vi "DifficultyValueChange.vi"(8 "error in (no error)":errorcluster, 11 "View in":refnum<class "View.lvclass">) -> (0 "error out":errorcluster, 3 "View out":refnum<class "View.lvclass">)   [LabVIEW 2024, in "GUI.lvlib" / "View.lvclass"]
uses:
  View.lvclass
  TypeDefs/Settings.ctl
  View.lvclass/View.ctl
  Controller/Controller.lvclass
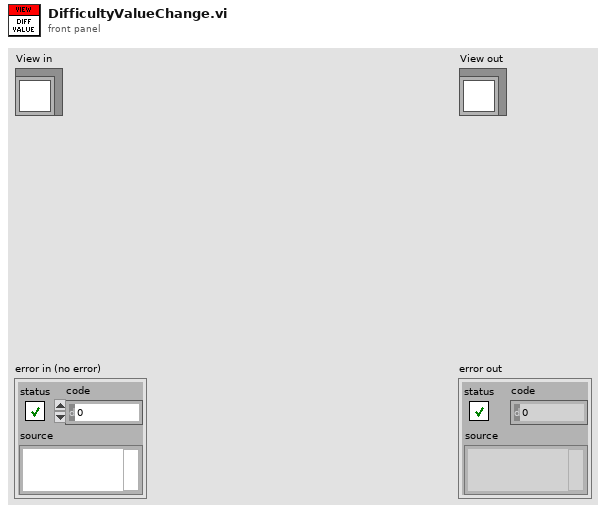
[diagram p1: front panel]
types:
  T1 = typedef "Settings.ctl" = cluster{"Difficulty":i32}
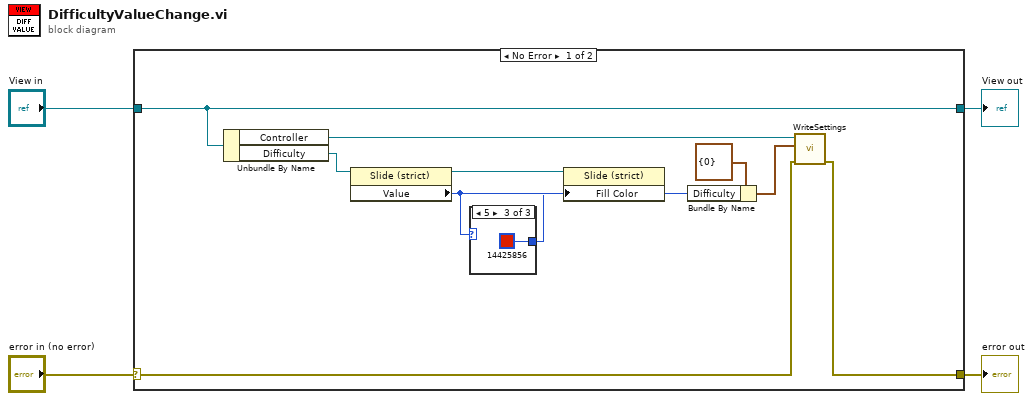
[diagram p0: block diagram]
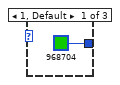
[diagram p2: hidden frame]
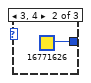
[diagram p3: hidden frame]
diagram:
  n1 = case shown="No Error" "error in (no error)" {
    selector: "error in (no error)" -> [w10 w19]
    tunnel: [w9 w19] -> w3
    tunnel: [w8 w18] -> w1
    tunnel: "View in" -> [w8 w18]
    frame No Error {
      n2 = Unbundle By Name(w8) -> ("Controller"=w14:refnum<class "Controller.lvclass">, "Difficulty"=w13:refnum<vi>)
      n3 = property class="Slide (strict)"(reference=w13) -> (reference out=w7:refnum<vi>, "Value"=w6:i32)  [unwired: 1 in, 1 out]
      n4 = case shown="5" w6 {
        tunnel: [u32 968704 u32 16771626 u32 14425856] -> w5
        frame 1, Default {
        }
        frame 3, 4 {
        }
        frame 5 {
        }
      }
      n5 = property class="Slide (strict)"(reference=w7, "Fill Color"=w5) -> ()  [unwired: 1 in, 2 out]
      n6 = Bundle By Name(cluster=T1 {"Difficulty"=0} ("Settings"), "Difficulty"=w6) -> (w11:T1)
      n7 = call "WriteSettings.vi"("error in (no error)"=w10, "Settings"=w11, "Controller in"=w14) -> ("error out"=w9:errorcluster)  [unwired: 7 in, 1 out]
    }
    frame Error {
    }
  }
  "error out" <- w3
  "View out" <- w1
